vi "get_frame_distribution.vi"(8 "error in (no error)":errorcluster, 11 "ImagingModeDL100901FlexTrajectory in":refnum<class "ImagingModeDL100901FlexTrajectory.lvclass">) -> (0 "error out":errorcluster, 1 "lines per frame":i32, 2 "number of frames":i32, 3 "ImagingModeDL100901FlexTrajectory out":refnum<class "ImagingModeDL100901FlexTrajectory.lvclass">)   [LabVIEW 2010, in "ImagingModeDL100901FlexTrajectory.lvclass"]
uses:
  ImagingModeDL100901FlexTrajectory.lvclass
  ImagingModeDL100901FlexTrajectory.lvclass/ImagingModeDL100901FlexTrajectory.ctl
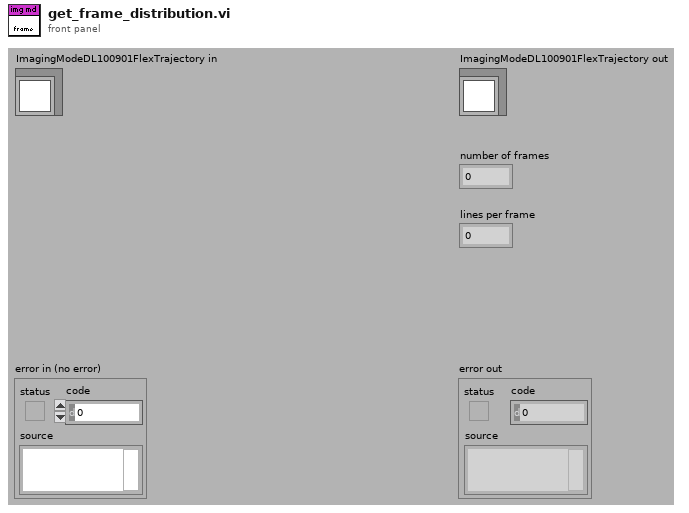
[diagram p1: front panel]
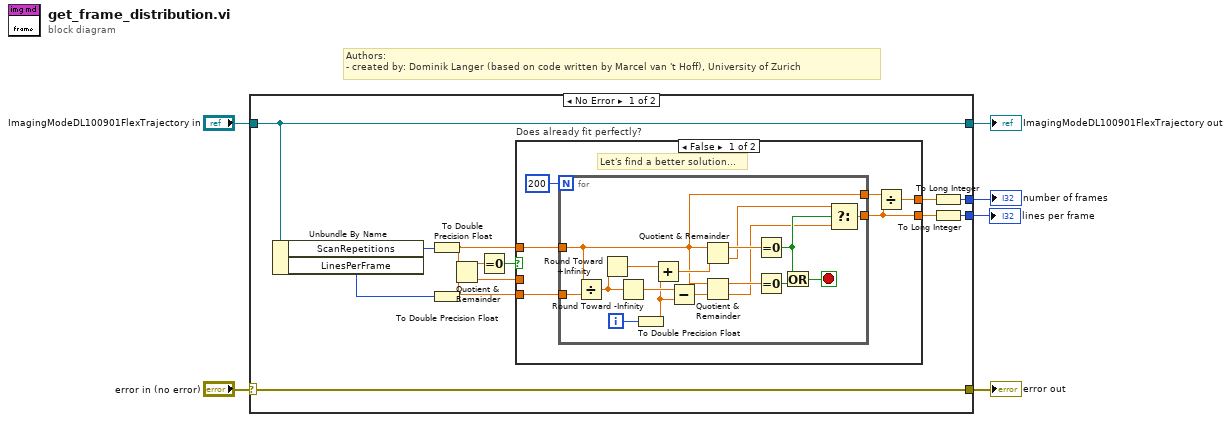
[diagram p0: block diagram]
diagram:
  # "Authors: \n- created by: Dominik Langer (based on code written by Marcel van 't Hoff), University of Zurich"
  n1 = case shown="No Error" "error in (no error)" {
    selector: "error in (no error)" -> [w19 w46]
    tunnel: [w19 w46] -> w5
    tunnel: [w11 w45] -> w3
    tunnel: "ImagingModeDL100901FlexTrajectory in" -> [w11 w45]
    tunnel: [w8 _] -> w2
    tunnel: [w7 _] -> w1
    frame No Error {
      n2 = Unbundle By Name(w11) -> ("ScanRepetitions"=w10:i32, "LinesPerFrame"=w9:i32)
      n3 = To Double Precision Float(number=w10) -> (double precision float=w13:dbl)
      n4 = To Double Precision Float(number=w9) -> (double precision float=w14:dbl)
      n5 = Quotient & Remainder(x=w13, y=w14) -> (x-y*floor(x/y)=w15:dbl, floor(x/y)=w12:dbl)
      n6 = Equal To 0?(x=w15) -> (x = 0?=w16:bool)
      n7 = case "Does already fit perfectly?" shown="False" w16 {
        tunnel: w14 -> [w25 w44]
        tunnel: w13 -> [w24 _]
        tunnel: [w20 w43] -> w17
        tunnel: [w21 w44] -> w18
        tunnel: w12 -> [_ w43]
        frame False {
          # "Let's find a better solution..."
          n8 = for {
            N: 200 -> [_]
            tunnel: w25 -> [w42]
            tunnel: w24 -> [w26]
            tunnel: [w27] -> w21
            tunnel: [w26] -> w22
            i -> [w32]
            stop <- w35 stop-if-true
            n9 = Divide(x=w26, y=w42) -> (x/y=w41:dbl)
            n10 = Round Toward +Infinity(x=w41) -> (ceil(x): smallest int >= x=w40:dbl)
            n11 = Round Toward -Infinity(1:w41) -> (0:w39:dbl)
            n12 = To Double Precision Float(number=w32) -> (double precision float=w31:dbl)
            n13 = Add(x=w40, y=w31) -> (x+y=w34:dbl)
            n14 = Subtract(x=w39, y=w31) -> (x-y=w33:dbl)
            n15 = Quotient & Remainder(x=w26, y=w34) -> (x-y*floor(x/y)=w38:dbl, floor(x/y)=w29:dbl)
            n16 = Quotient & Remainder(x=w26, y=w33) -> (x-y*floor(x/y)=w37:dbl, floor(x/y)=w28:dbl)
            n17 = Equal To 0?(x=w38) -> (x = 0?=w30:bool)
            n18 = Equal To 0?(x=w37) -> (x = 0?=w36:bool)
            n19 = Or(x=w30, y=w36) -> (x .or. y?=w35:bool)
            n20 = Select(t=w29, s=w30, f=w28) -> (s? t:f=w27:dbl)
          }
          n21 = Divide(x=w22, y=w21) -> (x/y=w20:dbl)
        }
        frame True {
        }
      }
      n22 = To Long Integer(number=w17) -> (32bit integer=w8:i32)
      n23 = To Long Integer(number=w18) -> (32bit integer=w7:i32)
    }
    frame Error {
    }
  }
  "error out" <- w5
  "ImagingModeDL100901FlexTrajectory out" <- w3
  "number of frames" <- w2
  "lines per frame" <- w1
